vi "Test SG08.vi"() -> ()   [LabVIEW 2009, in "POLARIS BME DG.lvlib"]
uses:
  LV-BME Interface/ChnlSettings.ctl
  LV-BME Interface/BME_DG_TriggerSettings.ctl
  LV-BME Interface/ClockSource.ctl
  DG Classes/BME_DG_G08/G08TriggerSettings.ctl
  DG Classes/BME_DG_System/BME_DG_System.lvclass
  DG Classes/BME_DG_G08_Chnl/BME_DG_G08_Chnl.lvclass
  DG Classes/BME_DG_G08/BME_DG_G08.lvclass
  DG Classes/BME_DG_Chnl/BME_DG_Chnl.lvclass
  DG Classes/BME_DG_Base/BME_DG_Base.lvclass
  POLARIS BME DG.lvlib
panel:
  in  "G08Settings":T1={"Gate Terminate"=TRUE, "Gate Level"=1.0, "Gate Delay (µs)"=0.0, "Step Back Time (µs)"=0.0, "Burst Counter"=0} {"Step Back Time (µs)" min=0.0 format="%.6f"; "Gate Delay (µs)" format="%.3f"; "Gate Level" min=-2.5 max=2.5 format="%.3g"}
  in  "V2 Trigger Settings":T2={"Gate Type"=TRUE, "Synchronize Gate"=FALSE, "Force Trigger (µs)"=0.0, "MS Bus"=1} {"MS Bus" format="%04x" items=["Local Primary"=1, "Local Secondary"=2, "Local Force"=4, "Resynchronize"=8, "Master Primary"=16, "Master Secondary"=32, "Master Force"=64, "System Clock"=128, "Delay Clock"=256, "Inhibit Local"=512, "Start Local"=1024, "Start Bus"=2048, "Step Back Local"=4096, "Step Back Bus"=8192, "Enable From E"=65536, "Enable From F"=131072, "Enable From Bus"=262144]; "Force Trigger (µs)" min=0.0 format="%.6f"}
  in  "SetDelay":bool=TRUE
  in  "UpdateChnl 2":bool=TRUE
  in  "ChnlParameter":T4 {"ChnParam2write"."Delay (µs)" min=0.0 max=100000000.0 format="%.5f"}
  out "Counts":i32
  in  "Acknowledge Interrupts":bool=TRUE
  out "TriggerCounters":i32[](array[numeric])
  out "Interrupts":u32[](array[numeric]) format="%b"
  in  "ClockSource Master":T5=1 items=["Internal Oscillator"=1, "External Trigger"=2, "Trigger & Oscillator"=3, "MasterSlave Bus"=4]
  in  "Trigger Settings SG02P2":T6={"InputTerminated?"=FALSE, "InternalClockPeriode(µs)"=1000000.0, "TriggerLevel"=1.25, "PresetValue"=0, "DivideBy"=1, "Clock Source"=1, "Gate Divider"=1, "PositiveGate?"=TRUE, "InternalTrigger?"=TRUE, "InternalArm?"=FALSE, "SWTrigger?"=FALSE, "RisingEdge?"=FALSE, "StopOnPreset?"=FALSE, "ResetWhenDone?"=TRUE, "TriggerEnabled?"=TRUE} {"Gate Divider" min=1 max=1000000; "Clock Source" items=["Internal Oscillator"=1, "External Trigger"=2, "Trigger & Oscillator"=3]; "InternalClockPeriode(µs)" format="%#_11g"}
  out "RemainingTriggers":T7(array[cluster])=[[{"Time Stamp"=timestamp(3416308194.6875 s since 1904-01-01), "Numeric"=-64}, {"Time Stamp"=timestamp(3416308194.6875 s since 1904-01-01), "Numeric"=4}, {"Time Stamp"=timestamp(3416308194.6875 s since 1904-01-01), "Numeric"=-64}, {"Time Stamp"=timestamp(3416308194.6875 s since 1904-01-01), "Numeric"=-64}], [{"Time Stamp"=timestamp(3416308194.6875 s since 1904-01-01), "Numeric"=-64}, {"Time Stamp"=timestamp(3416308194.6875 s since 1904-01-01), "Numeric"=-64}, {"Time Stamp"=timestamp(3416308194.6875 s since 1904-01-01), "Numeric"=-64}, {"Time Stamp"=timestamp(3416308194.6875 s since 1904-01-01), "Numeric"=-64}], [{"Time Stamp"=timestamp(3416308194.6875 s since 1904-01-01), "Numeric"=-64}, {"Time Stamp"=timestamp(3416308194.6875 s since 1904-01-01), "Numeric"=-64}, {"Time Stamp"=timestamp(3416308194.6875 s since 1904-01-01), "Numeric"=-64}, {"Time Stamp"=timestamp(3416308194.6875 s since 1904-01-01), "Numeric"=-64}]] {"Time Stamp" format="%<%I:%M:%S%3u %p>T"}
  in  "stop 2":bool=TRUE
  in  "ReadStatus":bool=TRUE
  in  "Activate":bool
  in  "UpdateChnl":bool=TRUE
  in  "TriggerModulo":u32=4
  out "Modulo Settings":u32[](array[numeric])
  out "Chnls":T3[](array[typedef])=[{" Delay (µs)"=0.0, "On? (false)"=TRUE, "PositiveVoltage?"=TRUE, "50OhmTerminated? "=TRUE, "25OhmOutput?"=FALSE}, {" Delay (µs)"=0.0, "On? (false)"=TRUE, "PositiveVoltage?"=TRUE, "50OhmTerminated? "=TRUE, "25OhmOutput?"=FALSE}, {" Delay (µs)"=0.0, "On? (false)"=TRUE, "PositiveVoltage?"=TRUE, "50OhmTerminated? "=TRUE, "25OhmOutput?"=FALSE}] {"Delay (µs)" min=0.0 max=100000000.0 format="%.5f"}
  in  "Selected Chnl":u16(ring) items=["S08P1_ChnlA", "S08P1_ChnlB", "S08P1_ChnlC", "S08P1_ChnlD", "S08P1_ChnlE", "S08P1_ChnlF"]
  in  "Selected Card":u16(ring)=1 items=["S08P1"]
  in  "STOP":bool=TRUE
  in  "ChnParam2write":T3={" Delay (µs)"=0.0, "On? (false)"=TRUE, "PositiveVoltage?"=TRUE, "50OhmTerminated? "=TRUE, "25OhmOutput?"=FALSE} {"Delay (µs)" min=0.0 max=100000000.0 format="%.5f"}
  # "INIT Values"
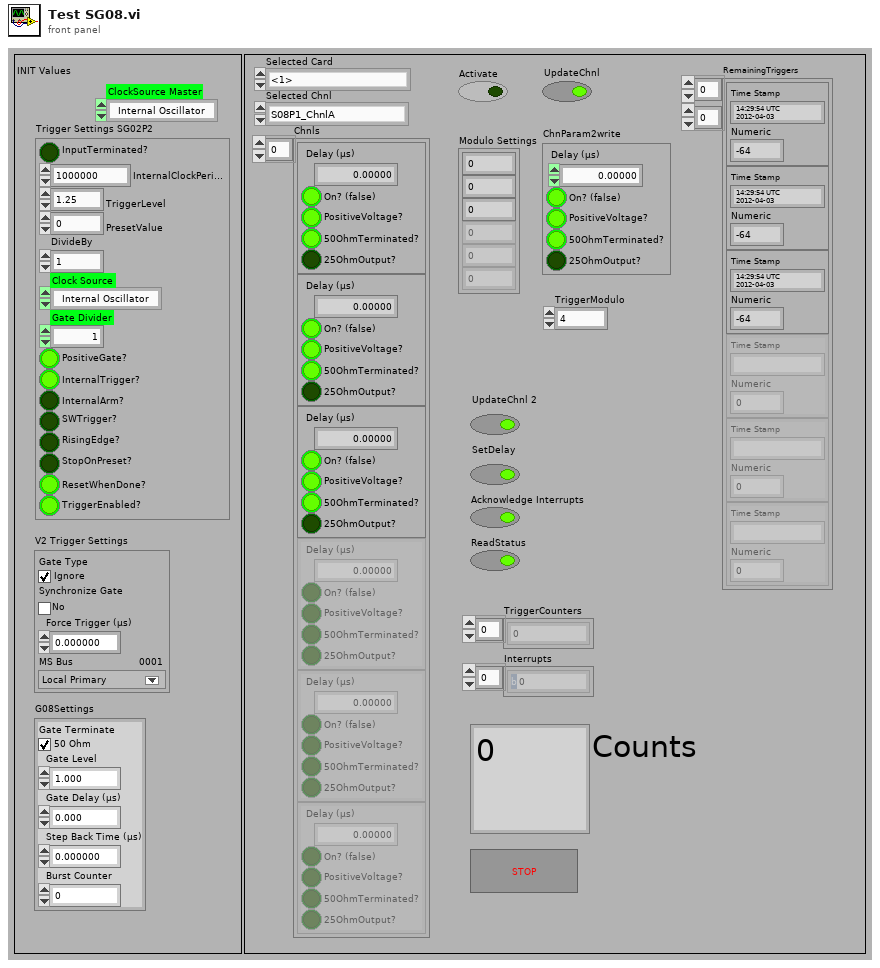
[diagram p1: front panel]
types:
  T1 = typedef "POLARIS BME DG.lvlib/BME_DG_G08.lvclass/G08TriggerSettings.ctl" = cluster{"Gate Terminate":bool, "Gate Level":dbl, "Gate Delay (µs)":dbl, "Step Back Time (µs)":dbl, "Burst Counter":u32}
  T2 = cluster{"Gate Type":bool, "Synchronize Gate":bool, "Force Trigger (µs)":dbl, "MS Bus":u32}
  T3 = typedef "POLARIS BME DG.lvlib/ChnlSettings.ctl" = cluster{" Delay (µs)":dbl, "On? (false)":bool, "PositiveVoltage?":bool, "50OhmTerminated? ":bool, "25OhmOutput?":bool}
  T4 = cluster{"ChnlName":string, "ChnParam2write":T3, "TriggerModulo":u32}
  T5 = typedef "POLARIS BME DG.lvlib/ClockSource.ctl" = i32
  T6 = typedef "POLARIS BME DG.lvlib/BME_DG_TriggerSettings.ctl" = cluster{"InputTerminated?":bool, "InternalClockPeriode(µs)":dbl, "TriggerLevel":dbl, "PresetValue":i32, "DivideBy":i32, "Clock Source":u32, "Gate Divider":i32, "PositiveGate?":bool, "InternalTrigger?":bool, "InternalArm?":bool, "SWTrigger?":bool, "RisingEdge?":bool, "StopOnPreset?":bool, "ResetWhenDone?":bool, "TriggerEnabled?":bool}
  T7 = cluster{"Time Stamp":timestamp, "Numeric":i32}[][]
  T8 = enum8{"Enabled", "Disabled", "Disabled and Grayed Out"}
  T9 = cluster{"ChnlName":string, "ChnParam2write":T3, "TriggerModulo":u32}[]
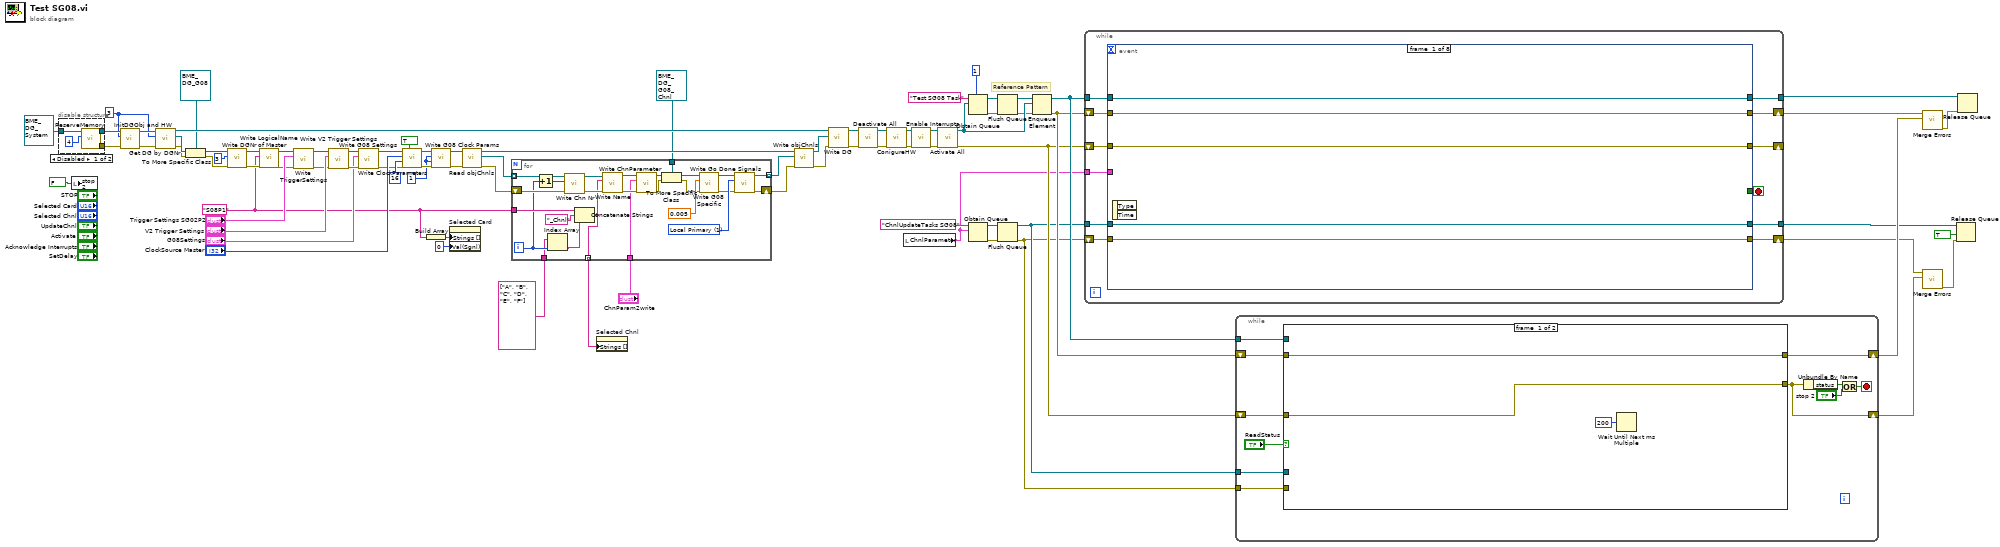
[diagram p0: block diagram]
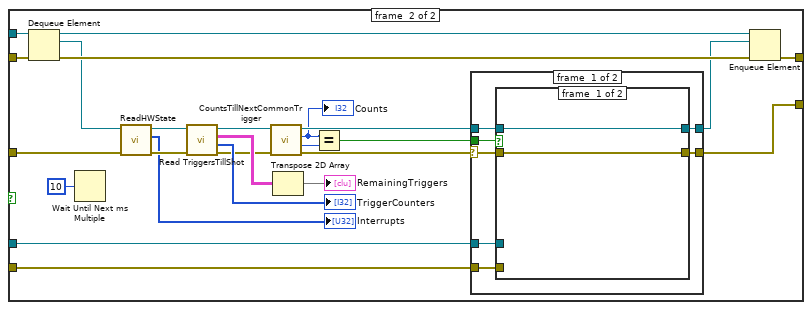
[diagram p3: hidden frame]
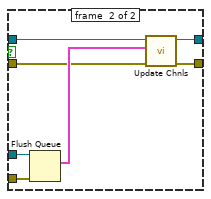
[diagram p4: hidden frame]
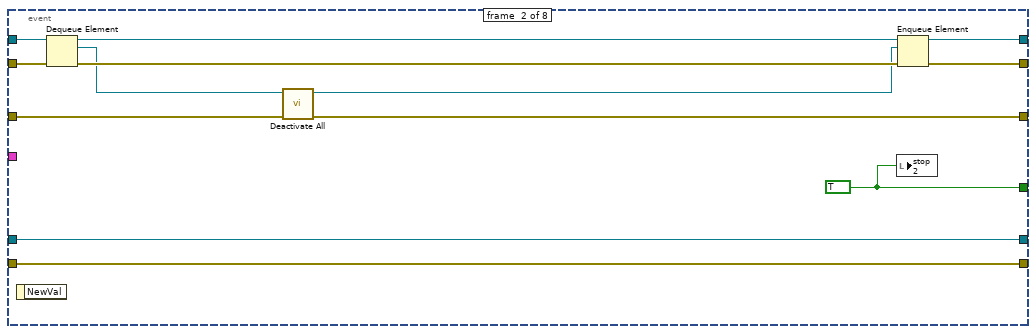
[diagram p6: hidden frame]
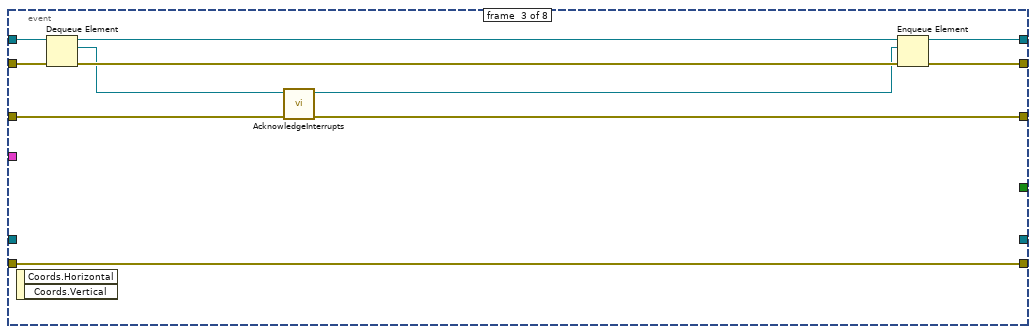
[diagram p7: hidden frame]
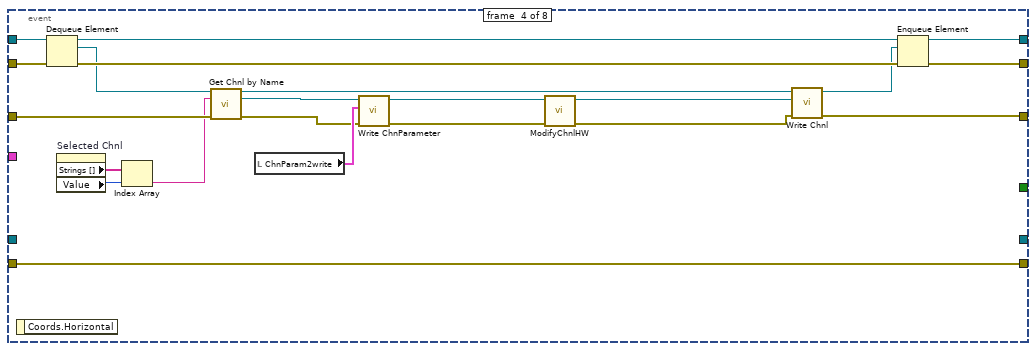
[diagram p8: hidden frame]
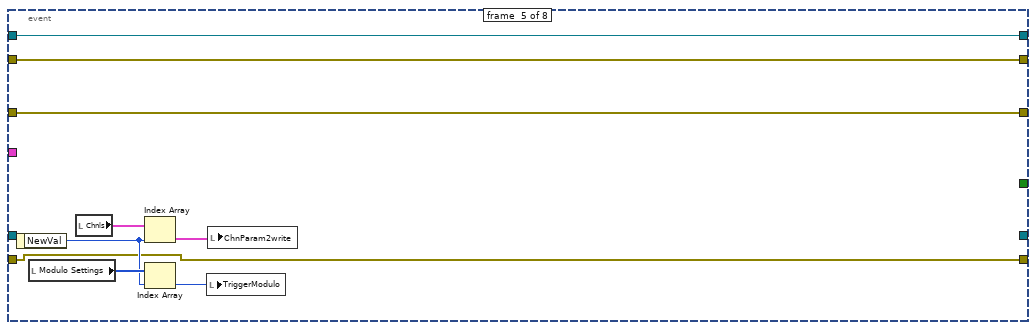
[diagram p9: hidden frame]
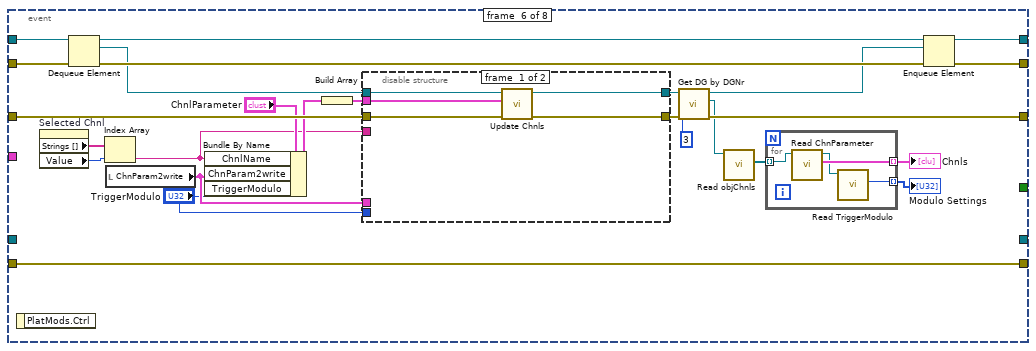
[diagram p10: hidden frame]
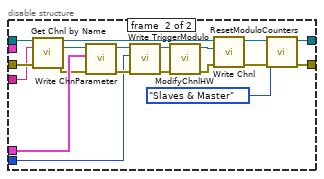
[diagram p11: hidden frame]
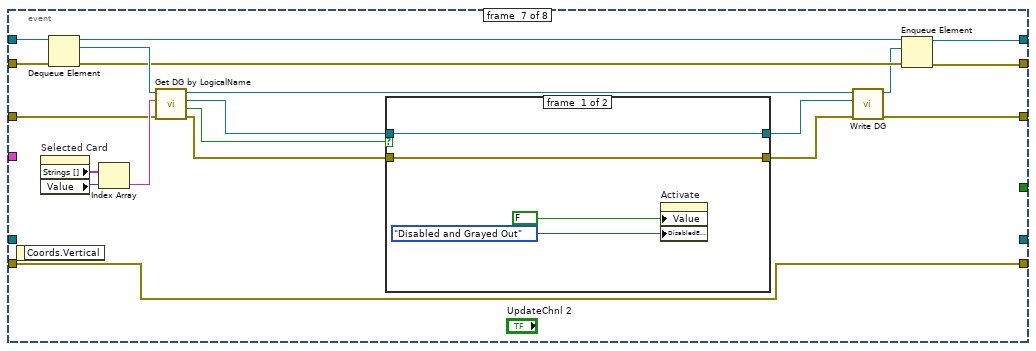
[diagram p12: hidden frame]
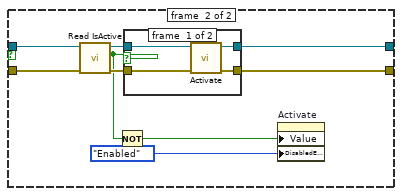
[diagram p13: hidden frame]
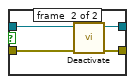
[diagram p14: hidden frame]
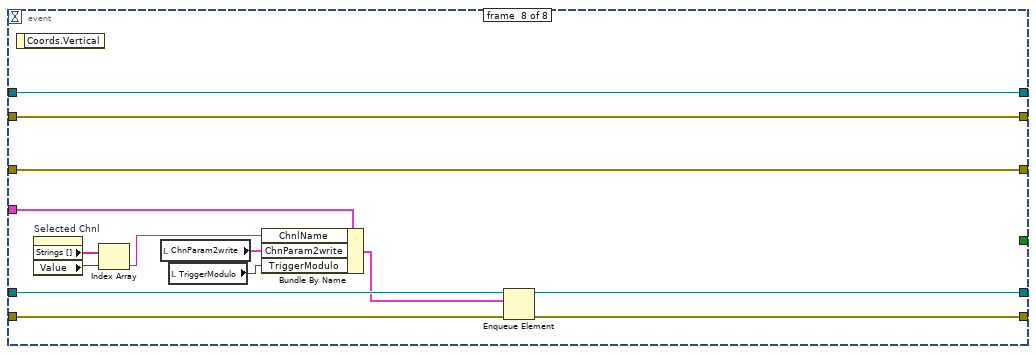
[diagram p15: hidden frame]
diagram:
  w19 = 3 ("DGNr")
  w25 = "S08P1"
  w40 = u32 1 ("Trigger Divider")
  # "Reference Pattern"
  n1 = disable-structure shown="Disabled" {
    disable-tunnel: refnum<class "BME_DG_System.lvclass"> refnum ("BME_DG_System.lvclass") -> [w86 w87]
    disable-tunnel: [w85 w87] -> w22
    disable-tunnel: [w84 _] -> w21
    frame #0 {
      n2 = call "ReserveMemory.vi"("#DGs"=4, "BME_DG_System in"=w86) -> ("error out"=w84:errorcluster, "BME_DG_System out"=w85:refnum<class "BME_DG_System.lvclass">)  [unwired: 8 in]
    }
    frame #1 {
    }
  }
  n3 = local write "stop 2"(FALSE ("stop 2")) -> ()
  n4 = call "InitDGObj and HW.vi"("error out"=w21, "DGNr"=w19, "BME_DG_System in"=w22) -> ("error IO"=w18:errorcluster, "BME_DG_System Out"=w20:refnum<class "BME_DG_System.lvclass">)  [unwired: 3 in]
  n5 = call "Get DG by DGNr.vi"("error in (no error)"=w18, "DG Nr."=w19, "BME_DG_System in"=w20) -> ("error out"=w13:errorcluster, "BME_DG_Base.lvclass"=w15:refnum<class "BME_DG_Base.lvclass">, "BME_DG_System out"=w17:refnum<class "BME_DG_System.lvclass">)  [unwired: 5 in, 1 out]
  n6 = To More Specific Class(target class=refnum<class "BME_DG_G08.lvclass"> refnum ("BME_DG_G08.lvclass"), reference=w15, error in=w13) -> (specific class reference=w14:refnum<class "BME_DG_G08.lvclass">, error out=w12:errorcluster)
  n7 = call-dynamic "Write DGNr of Master.vi"("error in (no error)"=w12, "DGNr of Master"=3, "BME_DG_Base in"=w14) -> ("error out"=w27:errorcluster, "BME_DG_Base out"=w28:refnum<class "BME_DG_G08.lvclass">)  [unwired: 7 in]
  n8 = call "Write LogicalName.vi"("error in (no error)"=w27, "LogicalName"=w25, "BME_DG_Base in"=w28) -> ("error out"=w9:errorcluster, "BME_DG_Base out"=w8:refnum<class "BME_DG_G08.lvclass">)  [unwired: 7 in]
  n9 = call-dynamic "Write TriggerSettings.vi"("error in (no error)"=w9, "Trigger Settings"="Trigger Settings SG02P2", "BME_DG_Base in"=w8) -> ("error out"=w10:errorcluster, "BME_DG_Base out"=w11:refnum<class "BME_DG_G08.lvclass">)  [unwired: 7 in]
  n10 = call-dynamic "Write V2 Trigger Settings.vi"("error in (no error)"=w10, "V2 Trigger Settings"="V2 Trigger Settings", "BME_DG_G05 in"=w11) -> ("error out"=w46:errorcluster, "BME_DG_G05 out"=w47:refnum<class "BME_DG_G08.lvclass">)  [unwired: 7 in]
  n11 = call-dynamic "Write G08 Settings.vi"("error in (no error)"=w46, "G08Settings"="G08Settings", "BME_DG_G08 in"=w47) -> ("error out"=w43:errorcluster, "BME_DG_G08 out"=w44:refnum<class "BME_DG_G08.lvclass">)  [unwired: 7 in]
  n12 = call-dynamic "Write ClockParameters.vi"("ClockEnable"=TRUE, "error in (no error)"=w43, "PrescalerCrystalOscilator"=u32 16, "ClockSource"="ClockSource Master", "BME_DG_Base in"=w44) -> ("error out"=w41:errorcluster, "BME_DG_Base out"=w42:refnum<class "BME_DG_G08.lvclass">)  [unwired: 5 in]
  n13 = Build Array(w25) -> (w24:string[])
  n14 = call-dynamic "Write G08 Clock Params.vi"("error in (no error)"=w41, "Trigger Multiplier"=w40, "Trigger Divider"=w40, "BME_DG_G08 in"=w42) -> ("error out"=w6:errorcluster, "BME_DG_G08 out"=w7:refnum<class "BME_DG_G08.lvclass">)  [unwired: 6 in]
  n15 = property on="Selected Card" class="Ring (strict)"("Strings []"=w24, "Val(Sgnl)"=u16 0 ("Value (Signaling)")) -> ()  [unwired: 2 in, 2 out]
  n16 = call-dynamic "Read objChnls.vi"("error in (no error)"=w6, "BME_DG_Base in"=w7) -> ("error out"=w34:errorcluster, "objChnls"=w35:refnum<class "BME_DG_Chnl.lvclass">[], "BME_DG_Base out"=w32:refnum<class "BME_DG_G08.lvclass">)  [unwired: 6 in, 1 out]
  n17 = for {
    tunnel: w35 -> [w107] mode=indexing
    shift-right: [w89] -> w30
    shift-left: w34 -> [w105]
    tunnel: w25 -> [w111]
    tunnel: "ChnParam2write" -> [w108]
    tunnel: [w91] -> w33 mode=indexing
    tunnel: string[] ["A", "B", "C", "D", "E", "F"] -> [w101]
    tunnel: refnum<class "BME_DG_G08_Chnl.lvclass"> refnum ("BME_DG_G08_Chnl.lvclass") -> [w92]
    tunnel: [w88] -> w1 mode=indexing
    i -> [w102]
    w98 = u32 1 items=["Local Primary"=1, "Local Secondary"=2, "Local Force"=4, "Resynchronize"=8, "Master Primary"=16, "Master Secondary"=32, "Master Force"=64, "System Clock"=128, "Delay Clock"=256, "Inhibit Local"=512, "Start Local"=1024, "Start Bus"=2048, "Step Back Local"=4096, "Step Back Bus"=8192, "From E"=65536, "From F"=131072, "From Bus"=262144] ("Go Signal")
    n18 = Increment(x=w102) -> (x+1=w103:i32)
    n19 = Index Array(array=w101, index=w102) -> (element=w100:string)
    n20 = call-dynamic "Write Chn Nr.vi"("error in (no error)"=w105, "Chn Nr"=w103, "BME_DG_Chnl in"=w107) -> ("error out"=w104:errorcluster, "BME_DG_Chnl out"=w106:refnum<class "BME_DG_Chnl.lvclass">)  [unwired: 7 in]
    n21 = Concatenate Strings(w111, "_Chnl" ("string"), w100) -> (w88:string)
    n22 = call-dynamic "Write Name.vi"("error in (no error)"=w104, "Name"=w88, "BME_DG_Chnl in"=w106) -> ("error out"=w109:errorcluster, "BME_DG_Chnl out"=w112:refnum<class "BME_DG_Chnl.lvclass">)  [unwired: 7 in]
    n23 = call-dynamic "Write ChnParameter.vi"("error in (no error)"=w109, "ChnParemater"=w108, "BME_DG_Chnl in"=w112) -> ("error out"=w90:errorcluster, "BME_DG_Chnl out"=w93:refnum<class "BME_DG_Chnl.lvclass">)  [unwired: 7 in]
    n24 = To More Specific Class(target class=w92, reference=w93, error in=w90) -> (specific class reference=w94:refnum<class "BME_DG_G08_Chnl.lvclass">, error out=w95:errorcluster)
    n25 = call-dynamic "Write G08 Specific.vi"("error in (no error)"=w95, "Pulse Width (µs)"=0.005, "BME_DG_G08_Chnl in"=w94) -> ("error out"=w97:errorcluster, "BME_DG_G08_Chnl out"=w96:refnum<class "BME_DG_G08_Chnl.lvclass">)  [unwired: 7 in]
    n26 = call-dynamic "Write Go Done Signals.vi"("error in (no error)"=w97, "Go Signal"=w98, "BME_DG_G05P2_Chnl in"=w96) -> ("error out"=w89:errorcluster, "BME_DG_G05P2_Chnl out"=w91:refnum<class "BME_DG_G08_Chnl.lvclass">)  [unwired: 7 in]
  }
  n27 = property on="Selected Chnl" class="Ring (strict)"("Strings []"=w1) -> ()  [unwired: 2 in, 2 out]
  n28 = call-dynamic "Write objChnls.vi"("error in (no error)"=w30, "objChnls"=w33, "BME_DG_Base in"=w32) -> ("error out"=w29:errorcluster, "BME_DG_Base out"=w31:refnum<class "BME_DG_G08.lvclass">)  [unwired: 7 in]
  n29 = call "Write DG.vi"("error in (no error)"=w29, "BME_DG_Base"=w31, "BME_DG_System in"=w17) -> ("error out"=w3:errorcluster, "BME_DG_System out"=w4:refnum<class "BME_DG_System.lvclass">)  [unwired: 7 in]
  n30 = call "Deactivate All.vi"("error in (no error)"=w3, "BME_DG_System in"=w4) -> ("error out"=w38:errorcluster, "BME_DG_System out"=w39:refnum<class "BME_DG_System.lvclass">)  [unwired: 8 in]
  n31 = call "ConigureHW.vi"("error in (no error)"=w38, "BME_DG_System in"=w39) -> ("error out"=w36:errorcluster, "BME_DG_System out"=w37:refnum<class "BME_DG_System.lvclass">)  [unwired: 8 in]
  n32 = local read "ChnlParameter"() -> (w60:T4)
  n33 = call "Enable Interrupts.vi"("error in (no error)"=w36, "BME_DG_System in"=w37) -> ("error out"=w64:errorcluster, "BME_DG_System out"=w65:refnum<class "BME_DG_System.lvclass">)  [unwired: 8 in]
  n34 = call "Activate All.vi"("error in (no error)"=w64, "BME_DG_System in"=w65) -> ("error out"=w72:errorcluster, "BME_DG_System out"=w79:refnum<class "BME_DG_System.lvclass">)  [unwired: 8 in]
  n35 = Obtain Queue(max queue size (-1, unlimited)=1, name (unnamed)="Test SG08 Task", element data type=w79) -> (queue out=w70:refnum<queue>, error out=w68:errorcluster)  [unwired: 2 in, 1 out]
  n36 = Obtain Queue(name (unnamed)="ChnlUpdateTasks SG08", element data type=w60) -> (queue out=w61:refnum<queue>, error out=w62:errorcluster)  [unwired: 3 in, 1 out]
  n37 = Flush Queue(queue=w70, error in (no error)=w68) -> (queue out=w69:refnum<queue>, error out=w67:errorcluster)  [unwired: 1 out]
  n38 = Flush Queue(queue=w61, error in (no error)=w62) -> (queue out=w57:refnum<queue>, error out=w56:errorcluster)  [unwired: 1 out]
  n39 = Enqueue Element(queue=w69, element=w79, error in (no error)=w67) -> (queue out=w78:refnum<queue>, error out=w77:errorcluster)  [unwired: 1 in, 1 out]
  n40 = while {
    shift-right: [w120] -> _
    shift-left: w72 -> [w122]
    shift-right: [w118] -> w74
    shift-left: w77 -> [w119]
    tunnel: w78 -> [w123]
    tunnel: [w121] -> w76
    tunnel: w57 -> [w117]
    tunnel: w60 -> [w116]
    tunnel: [w114] -> w59
    shift-right: [w113] -> w55
    shift-left: w56 -> [w115]
    stop <- w124 stop-if-true
    n41 = event shown="[5] \"UpdateChnl\": Mouse Down;  \"UpdateChnl\": Key Down" {
      selector: _ -> [_ _ _ _ _ _ _ _]
      dyn-events: _ -> [_ _ _ _ _ _ _ _]
      timeout: _ -> [_ _ _ _ _ _ _ _]
      tunnel: [_ w132 _ _ _ _ _ _] -> w124
      tunnel: w123 -> [w129 w139 w152 w174 w184 w208 w247 w293]
      tunnel: w122 -> [w128 w142 w144 w165 w183 w201 w255 w292]
      tunnel: [w129 w135 w148 w170 w184 w203 w241 w293] -> w121
      tunnel: [w128 w141 w145 w154 w183 w194 w248 w292] -> w120
      tunnel: w119 -> [w127 w138 w151 w173 w177 w206 w246 w289]
      tunnel: [w127 w136 w149 w171 w177 w204 w240 w289] -> w118
      tunnel: w117 -> [w126 w131 _ _ _ _ _ w284]
      tunnel: w116 -> [_ _ _ _ _ _ _ w288]
      tunnel: w115 -> [w125 w130 w143 w169 w176 w199 w239 w282]
      tunnel: [w126 w131 _ _ _ _ _ w281] -> w114
      tunnel: [w125 w130 w143 w169 w176 w199 w239 w280] -> w113
      event #0 {
        n42 = event-data() -> ()  [unwired: 1 in, 2 out]
      }
      event #1 {
        w132 = TRUE
        n43 = event-data() -> ()  [unwired: 1 in, 1 out]
        n44 = Dequeue Element(queue=w139, error in (no error)=w138) -> (queue out=w140:refnum<queue>, element=w133:refnum<class "BME_DG_System.lvclass">, error out=w137:errorcluster)  [unwired: 1 in, 1 out]
        n45 = call "Deactivate All.vi"("error in (no error)"=w142, "BME_DG_System in"=w133) -> ("error out"=w141:errorcluster, "BME_DG_System out"=w134:refnum<class "BME_DG_System.lvclass">)  [unwired: 8 in]
        n46 = local write "stop 2"(w132) -> ()
        n47 = Enqueue Element(queue=w140, element=w134, error in (no error)=w137) -> (queue out=w135:refnum<queue>, error out=w136:errorcluster)  [unwired: 1 in, 1 out]
      }
      event #2 {
        n48 = event-data() -> ()  [unwired: 1 in, 2 out]
        n49 = Dequeue Element(queue=w152, error in (no error)=w151) -> (queue out=w153:refnum<queue>, element=w147:refnum<class "BME_DG_System.lvclass">, error out=w150:errorcluster)  [unwired: 1 in, 1 out]
        n50 = call "AcknowledgeInterrupts.vi"("error in (no error)"=w144, "BME_DG_System in"=w147) -> ("error out"=w145:errorcluster, "BME_DG_System out"=w146:refnum<class "BME_DG_System.lvclass">)  [unwired: 8 in]
        n51 = Enqueue Element(queue=w153, element=w146, error in (no error)=w150) -> (queue out=w148:refnum<queue>, error out=w149:errorcluster)  [unwired: 1 in, 1 out]
      }
      event #3 {
        n52 = event-data() -> ()  [unwired: 1 in, 1 out]
        n53 = Dequeue Element(queue=w174, error in (no error)=w173) -> (queue out=w175:refnum<queue>, element=w166:refnum<class "BME_DG_System.lvclass">, error out=w172:errorcluster)  [unwired: 1 in, 1 out]
        n54 = property on="Selected Chnl" class="Ring (strict)"() -> ("Strings []"=w167:string[], "Value"=w168:u16)  [unwired: 2 in, 2 out]
        n55 = Index Array(array=w167, index=w168) -> (element=w164:string)
        n56 = call "Get Chnl by Name.vi"("BME_DG_System in"=w166, "Chnl Name"=w164, "error in (no error)"=w165) -> ("BME_DG_System out"=w160:refnum<class "BME_DG_System.lvclass">, "BME_DG_Chnl"=w163:refnum<class "BME_DG_Chnl.lvclass">, "error out"=w161:errorcluster)  [unwired: 7 in, 3 out]
        n57 = local read "ChnParam2write"() -> (w162:T3)
        n58 = call-dynamic "Write ChnParameter.vi"("error in (no error)"=w161, "ChnParemater"=w162, "BME_DG_Chnl in"=w163) -> ("error out"=w157:errorcluster, "BME_DG_Chnl out"=w158:refnum<class "BME_DG_Chnl.lvclass">)  [unwired: 7 in]
        n59 = call-dynamic "ModifyChnlHW.vi"("error in (no error)"=w157, "BME_DG_Chnl in"=w158) -> ("error out"=w155:errorcluster, "BME_DG_Chnl out"=w156:refnum<class "BME_DG_Chnl.lvclass">)  [unwired: 8 in]
        n60 = call "Write Chnl.vi"("error in (no error)"=w155, "BME_DG_Chnl.lvclass"=w156, "BME_DG_System in"=w160) -> ("error out"=w154:errorcluster, "BME_DG_System out"=w159:refnum<class "BME_DG_System.lvclass">)  [unwired: 7 in]
        n61 = Enqueue Element(queue=w175, element=w159, error in (no error)=w172) -> (queue out=w170:refnum<queue>, error out=w171:errorcluster)  [unwired: 1 in, 1 out]
      }
      event #4 {
        n62 = event-data() -> ("NewVal"=w180:u16)  [unwired: 1 in]
        n63 = local read "Modulo Settings"() -> (w181:u32[])
        n64 = local read "Chnls"() -> (w182:T3[])
        n65 = Index Array(array=w182, index=w180) -> (element=w179:T3)
        n66 = Index Array(array=w181, index=w180) -> (element=w178:u32)
        n67 = local write "TriggerModulo"(w178) -> ()
        n68 = local write "ChnParam2write"(w179) -> ()
      }
      event #5 {
        n69 = event-data() -> ()  [unwired: 1 in, 1 out]
        n70 = property on="Selected Chnl" class="Ring (strict)"() -> ("Strings []"=w210:string[], "Value"=w209:u16)  [unwired: 2 in, 2 out]
        n71 = Dequeue Element(queue=w208, error in (no error)=w206) -> (queue out=w207:refnum<queue>, element=w202:refnum<class "BME_DG_System.lvclass">, error out=w205:errorcluster)  [unwired: 1 in, 1 out]
        n72 = Index Array(array=w210, index=w209) -> (element=w187:string)
        n73 = local read "ChnParam2write"() -> (w186:T3)
        n74 = Bundle By Name(cluster="ChnlParameter", "ChnlName"=w187, "ChnParam2write"=w186, "TriggerModulo"="TriggerModulo") -> (w188:T4)
        n75 = Build Array(w188) -> (w198:T9)
        n76 = disable-structure shown="Enabled" {
          disable-tunnel: w202 -> [w215 w234]
          disable-tunnel: w201 -> [w214 w233]
          disable-tunnel: w198 -> [w213 _]
          disable-tunnel: [w212 w219] -> w197
          disable-tunnel: [w211 w217] -> w195
          disable-tunnel: w187 -> [_ w232]
          disable-tunnel: w186 -> [_ w229]
          disable-tunnel: "TriggerModulo" -> [_ w221]
          frame #0 {
            n77 = call "Update Chnls.vi"("error in (no error)"=w214, "ChnlSettings"=w213, "BME_DG_System in"=w215) -> ("error out"=w211:errorcluster, "BME_DG_System out"=w212:refnum<class "BME_DG_System.lvclass">)  [unwired: 7 in]
          }
          frame #1 {
            n78 = call "Get Chnl by Name.vi"("BME_DG_System in"=w234, "Chnl Name"=w232, "error in (no error)"=w233) -> ("BME_DG_System out"=w231:refnum<class "BME_DG_System.lvclass">, "BME_DG_Chnl"=w230:refnum<class "BME_DG_Chnl.lvclass">, "error out"=w226:errorcluster)  [unwired: 7 in, 3 out]
            n79 = call-dynamic "Write ChnParameter.vi"("error in (no error)"=w226, "ChnParemater"=w229, "BME_DG_Chnl in"=w230) -> ("error out"=w227:errorcluster, "BME_DG_Chnl out"=w228:refnum<class "BME_DG_Chnl.lvclass">)  [unwired: 7 in]
            n80 = call-dynamic "Write TriggerModulo.vi"("error in (no error)"=w227, "TriggerModulo"=w221, "BME_DG_G05_Chnl in"=w228) -> ("error out"=w224:errorcluster, "BME_DG_G05_Chnl out"=w225:refnum<class "BME_DG_Chnl.lvclass">)  [unwired: 7 in]
            n81 = call-dynamic "ModifyChnlHW.vi"("error in (no error)"=w224, "BME_DG_Chnl in"=w225) -> ("error out"=w223:errorcluster, "BME_DG_Chnl out"=w222:refnum<class "BME_DG_Chnl.lvclass">)  [unwired: 8 in]
            n82 = call "Write Chnl.vi"("error in (no error)"=w223, "BME_DG_Chnl.lvclass"=w222, "BME_DG_System in"=w231) -> ("error out"=w218:errorcluster, "BME_DG_System out"=w220:refnum<class "BME_DG_System.lvclass">)  [unwired: 7 in]
            n83 = call "ResetModuloCounters.vi"("error in (no error)"=w218, "Enum"=enum16{"Slaves only", "Slaves & Master"}."Slaves & Master", "BME_DG_System in"=w220) -> ("error out"=w217:errorcluster, "BME_DG_System out"=w219:refnum<class "BME_DG_System.lvclass">)  [unwired: 7 in]
          }
        }
        n84 = call "Get DG by DGNr.vi"("error in (no error)"=w195, "DG Nr."=3, "BME_DG_System in"=w197) -> ("error out"=w194:errorcluster, "BME_DG_Base.lvclass"=w193:refnum<class "BME_DG_Base.lvclass">, "BME_DG_System out"=w196:refnum<class "BME_DG_System.lvclass">)  [unwired: 5 in, 1 out]
        n85 = call-dynamic "Read objChnls.vi"("BME_DG_Base in"=w193) -> ("objChnls"=w192:refnum<class "BME_DG_Chnl.lvclass">[])  [unwired: 7 in, 3 out]
        n86 = for {
          tunnel: w192 -> [w238] mode=indexing
          tunnel: [w237] -> w191 mode=indexing
          tunnel: [w235] -> w189 mode=indexing
          n87 = call-dynamic "Read ChnParameter.vi"("BME_DG_Chnl in"=w238) -> ("ChnParemater"=w237:T3, "BME_DG_Chnl out"=w236:refnum<class "BME_DG_Chnl.lvclass">)  [unwired: 5 in, 4 out]
          n88 = call-dynamic "Read TriggerModulo.vi"("BME_DG_Chnl in"=w236) -> ("TriggerModulo"=w235:i32)  [unwired: 8 in, 2 out]
        }
        "Chnls" <- w191
        "Modulo Settings" <- w189
        n89 = Enqueue Element(queue=w207, element=w196, error in (no error)=w205) -> (queue out=w203:refnum<queue>, error out=w204:errorcluster)  [unwired: 1 in, 1 out]
      }
      event #6 {
        n90 = event-data() -> ()  [unwired: 1 in, 1 out]
        n91 = property on="Selected Card" class="Ring (strict)"() -> ("Strings []"=w258:string[], "Value"=w257:u16)  [unwired: 2 in, 2 out]
        n92 = Dequeue Element(queue=w247, error in (no error)=w246) -> (queue out=w244:refnum<queue>, element=w245:refnum<class "BME_DG_System.lvclass">, error out=w243:errorcluster)  [unwired: 1 in, 1 out]
        n93 = Index Array(array=w258, index=w257) -> (element=w256:string)
        n94 = call "Get DG by LogicalName.vi"("error in (no error)"=w255, "LogicalName"=w256, "BME_DG_System in"=w245) -> ("error out"=w253:errorcluster, "found?"=w249:bool, "BME_DG_Base.lvclass"=w254:refnum<class "BME_DG_Base.lvclass">, "BME_DG_System out"=w250:refnum<class "BME_DG_System.lvclass">)  [unwired: 5 in]
        n95 = case shown="True" w249 {
          tunnel: w254 -> [w262 w269]
          tunnel: w253 -> [w261 w267]
          tunnel: [w261 w271] -> w252
          tunnel: [w262 w270] -> w251
          frame #0 {
            n96 = property on="Activate" class="Bool (strict)"("Value"=FALSE ("Activate"), "DisabledEnum"=T8."Disabled and Grayed Out" ("Disabled")) -> ()  [unwired: 2 in, 2 out]
          }
          frame #1 {
            n97 = call-dynamic "Read IsActive.vi"("error in (no error)"=w267, "BME_DG_Base in"=w269) -> ("error out"=w266:errorcluster, "Active?"=w265:bool, "BME_DG_Base out"=w268:refnum<class "BME_DG_Base.lvclass">)  [unwired: 7 in]
            n98 = Not(x=w265) -> (.not. x?=w263:bool)
            n99 = case shown="True" w265 {
              tunnel: [w275 w277] -> w271
              tunnel: [w274 w278] -> w270
              tunnel: w268 -> [w273 w279]
              tunnel: w266 -> [w272 w276]
              frame #0 {
                n100 = call-dynamic "Activate.vi"("error in (no error)"=w272, "BME_DG_Base in"=w273) -> ("error out"=w275:errorcluster, "BME_DG_Base out"=w274:refnum<class "BME_DG_Base.lvclass">)  [unwired: 8 in]
              }
              frame #1 {
                n101 = call-dynamic "Deactivate.vi"("error in (no error)"=w276, "BME_DG_Base in"=w279) -> ("error out"=w277:errorcluster, "BME_DG_Base out"=w278:refnum<class "BME_DG_Base.lvclass">)  [unwired: 8 in]
              }
            }
            n102 = property on="Activate" class="Bool (strict)"("Value"=w263, "DisabledEnum"=T8."Enabled" ("Disabled")) -> ()  [unwired: 2 in, 2 out]
          }
        }
        n103 = call "Write DG.vi"("error in (no error)"=w252, "BME_DG_Base"=w251, "BME_DG_System in"=w250) -> ("error out"=w248:errorcluster, "BME_DG_System out"=w242:refnum<class "BME_DG_System.lvclass">)  [unwired: 7 in]
        n104 = Enqueue Element(queue=w244, element=w242, error in (no error)=w243) -> (queue out=w241:refnum<queue>, error out=w240:errorcluster)  [unwired: 1 in, 1 out]
      }
      event #7 {
        n105 = event-data() -> ()  [unwired: 1 in, 1 out]
        n106 = property on="Selected Chnl" class="Ring (strict)"() -> ("Strings []"=w290:string[], "Value"=w291:u16)  [unwired: 2 in, 2 out]
        n107 = Index Array(array=w290, index=w291) -> (element=w287:string)
        n108 = local read "ChnParam2write"() -> (w286:T3)
        n109 = local read "TriggerModulo"() -> (w285:u32)
        n110 = Bundle By Name(cluster=w288, "ChnlName"=w287, "ChnParam2write"=w286, "TriggerModulo"=w285) -> (w283:T4)
        n111 = Enqueue Element(queue=w284, element=w283, error in (no error)=w282) -> (queue out=w281:refnum<queue>, error out=w280:errorcluster)  [unwired: 1 in, 1 out]
      }
    }
  }
  n112 = while {
    tunnel: w78 -> [w301]
    shift-right: [w299] -> w73
    shift-left: w77 -> [w300]
    shift-right: [w296] -> w54
    shift-left: w72 -> [w298]
    tunnel: w57 -> [w295]
    tunnel: w56 -> [w294]
    stop <- w303 stop-if-true
    n113 = case shown="True" "ReadStatus" {
      tunnel: w301 -> [_ w330]
      tunnel: w300 -> [w306 w329]
      tunnel: [w306 w328] -> w299
      tunnel: w298 -> [w305 w326]
      tunnel: [w305 w312] -> w296
      tunnel: w295 -> [_ w316]
      tunnel: w294 -> [_ w315]
      frame #0 {
        n114 = Wait Until Next ms Multiple(millisecond multiple=u32 200) -> ()  [unwired: 1 out]
      }
      frame #1 {
        n115 = Dequeue Element(queue=w330, error in (no error)=w329) -> (queue out=w331:refnum<queue>, element=w327:refnum<class "BME_DG_System.lvclass">, error out=w332:errorcluster)  [unwired: 1 in, 1 out]
        n116 = Wait Until Next ms Multiple(millisecond multiple=u32 10) -> ()  [unwired: 1 out]
        n117 = call "ReadHWState.vi"("error in (no error)"=w326, "BME_DG_System in"=w327) -> ("error out"=w325:errorcluster, "Interrupts"=→"Interrupts":u32[], "BME_DG_System out"=w324:refnum<class "BME_DG_System.lvclass">)  [unwired: 7 in]
        n118 = call "Read TriggersTillShot.vi"("error in (no error)"=w325, "BME_DG_System in"=w324) -> ("error out"=w317:errorcluster, "TriggerCounters"=→"TriggerCounters":i32[], "RemainingTriggers"=w323:T7, "BME_DG_System out"=w318:refnum<class "BME_DG_System.lvclass">)  [unwired: 6 in]
        n119 = call "CountsTillNextCommonTrigger.vi"("error in (no error)"=w317, "BME_DG_System in"=w318) -> ("error out"=w314:errorcluster, "LeastCommonMult"=w309:i32, "CountsRemains"=w310:i32, "BME_DG_System out"=w313:refnum<class "BME_DG_System.lvclass">)  [unwired: 6 in]
        "Counts" <- w310
        n120 = Transpose 2D Array(2D array=w323) -> (transposed array=→"RemainingTriggers":T7)
        n121 = Equal?(x=w310, y=w309) -> (x = y?=w308:bool)
        n122 = case shown="No Error" w314 {
          selector: w314 -> [w336 w349]
          tunnel: w316 -> [w339 _]
          tunnel: w315 -> [w338 _]
          tunnel: w313 -> [w337 w350]
          tunnel: [w335 w349] -> w312
          tunnel: [w334 w350] -> w311
          tunnel: w308 -> [w333 _]
          frame #0 {
            n123 = case shown="True" w333 {
              tunnel: w339 -> [_ w348]
              tunnel: w338 -> [_ w347]
              tunnel: w337 -> [w341 w346]
              tunnel: w336 -> [w340 w344]
              tunnel: [w340 w343] -> w335
              tunnel: [w341 w342] -> w334
              frame #0 {
              }
              frame #1 {
                n124 = Flush Queue(queue=w348, error in (no error)=w347) -> (remaining elements=w345:T9)  [unwired: 2 out]
                n125 = call "Update Chnls.vi"("error in (no error)"=w344, "ChnlSettings"=w345, "BME_DG_System in"=w346) -> ("error out"=w343:errorcluster, "BME_DG_System out"=w342:refnum<class "BME_DG_System.lvclass">)  [unwired: 7 in]
              }
            }
          }
          frame #1 {
          }
        }
        n126 = Enqueue Element(queue=w331, element=w311, error in (no error)=w332) -> (error out=w328:errorcluster)  [unwired: 1 in, 2 out]
      }
    }
    n127 = Unbundle By Name(w296) -> ("status"=w302:bool)
    n128 = Or(x=w302, y="stop 2") -> (x .or. y?=w303:bool)
  }
  n129 = call <vilib>:"Merge Errors.vi"("error in 2 (no error)"=w73, "error in 1 (no error)"=w74) -> ("error out"=w75:errorcluster)  [unwired: 5 in]
  n130 = call <vilib>:"Merge Errors.vi"("error in 2 (no error)"=w54, "error in 1 (no error)"=w55) -> ("error out"=w53:errorcluster)  [unwired: 5 in]
  n131 = Release Queue(queue=w59, force destroy? (F)=TRUE, error in (no error)=w53) -> ()  [unwired: 3 out]
  n132 = Release Queue(queue=w76, error in (no error)=w75) -> ()  [unwired: 1 in, 3 out]
